vi "Get Axis Motion Status.vi"(4 "error in (no error)":errorcluster, 6 "Axis (1)":i32=1 min=1 max=3, 7 "VISA resource name":refnum<visa-resource-name>) -> (0 "error out":errorcluster, 2 "Motion Done":bool, 3 "VISA resource name out":refnum<visa-resource-name>)   [LabVIEW 2020, in "Newport ESP301.lvlib"]
doc: "Reads the motion status for the specified axis. This command can be used to monitor Homing, absolute and relative displacement move completion status."
uses:
  Newport ESP301.lvlib
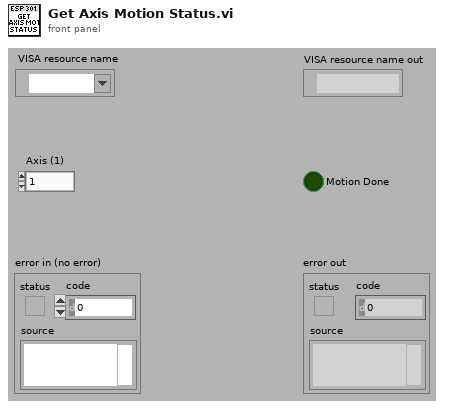
[diagram p1: front panel]
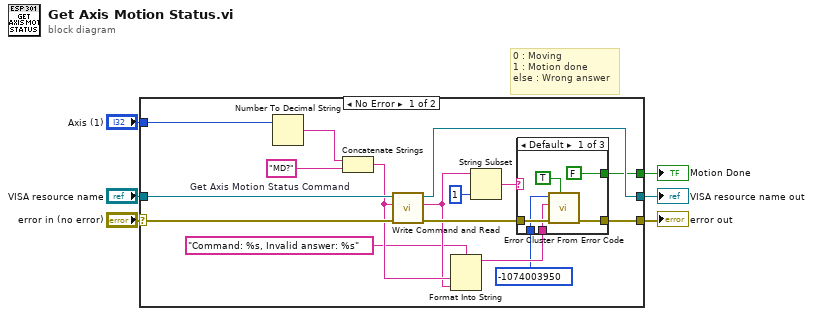
[diagram p0: block diagram]
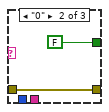
[diagram p2: hidden frame]
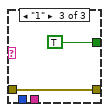
[diagram p3: hidden frame]
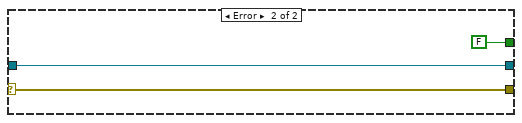
[diagram p4: hidden frame]
diagram:
  # "0 : Moving\n1 : Motion done\nelse : Wrong answer"
  n1 = case shown="No Error" "error in (no error)" {
    selector: "error in (no error)" -> [w21 w35]
    tunnel: [w14 w35] -> w5
    tunnel: "VISA resource name" -> [w22 w34]
    tunnel: [w13 w34] -> w3
    tunnel: "Axis (1)" -> [w19 _]
    tunnel: [w12 FALSE ("Motion Done")] -> w1
    frame No Error {
      w18 = "MD?"  # Get Axis Motion Status Command
      n2 = Number To Decimal String(number=w19) -> (decimal integer string=w20:string)  [unwired: 1 in]
      n3 = Concatenate Strings(w20, w18) -> (w11:string)
      n4 = call "Write Command and Read.vi"("error in (no error)"=w21, "Command"=w11, "VISA resource name"=w22) -> ("error out"=w15:errorcluster, "Returned string"=w10:string, "VISA resource name out"=w13:refnum<visa-resource-name>)  [unwired: 4 in]
      n5 = Format Into String(format string="Command: %s, Invalid answer: %s" ("error message (\"\")"), w11, w10) -> (resulting string=w8:string)  [unwired: 2 in, 1 out]
      n6 = String Subset(string=w10, length (rest)=1 ("longueur (reste)")) -> (substring=w16:string)  [unwired: 1 in]
      n7 = case shown="Default" w16 {
        tunnel: w15 -> [w25 w30 w32]
        tunnel: [w27 w30 w32] -> w14
        tunnel: [FALSE ("Motion Done") FALSE ("Motion Done") TRUE ("Motion Done")] -> w12
        tunnel: w8 -> [w24 _ _]
        tunnel: -1074003950 ("error code (0)") -> [w23 _ _]
        frame Default {
          n8 = call <vilib>:"Error Cluster From Error Code.vi"("show call chain? (False)"=TRUE, "error in (no error)"=w25, "error message (\"\")"=w24, "error code (0)"=w23) -> ("error out"=w27:errorcluster)  [unwired: 5 in]
        }
        frame "0" {
        }
        frame "1" {
        }
      }
    }
    frame Error {
    }
  }
  "error out" <- w5
  "VISA resource name out" <- w3
  "Motion Done" <- w1
